vi "Resistance Test_ver2_3.vi"(0 "DMM ref in":refnum<visa-resource-name>, 1 "Measure\nMax Voltage":dbl=100.0, 2 "Resistance Test REF":refnum<vi>, 3 "Resistance Test Stop REF":refnum<vi>, 5 "PSU setting":T1, 7 "Channel  Count":i32, 9 "ESP32 ref in":refnum<visa-resource-name>="COM4", 11 "ESP32 error in":errorcluster, 12 "Wait Current Stable Period":u32, 13 "Manual Trigger Delay (1 s)":dbl=1.0, 14 "Current Sense \nResitance Array":dbl[](array[numeric])) -> (10 "ESP32 ref out":refnum<visa-resource-name>, 15 "ESP32 error out":errorcluster)   [LabVIEW 2023]
uses:
  <instrlib>/Agilent 3446X Series/Agilent 3446X Series.lvlib
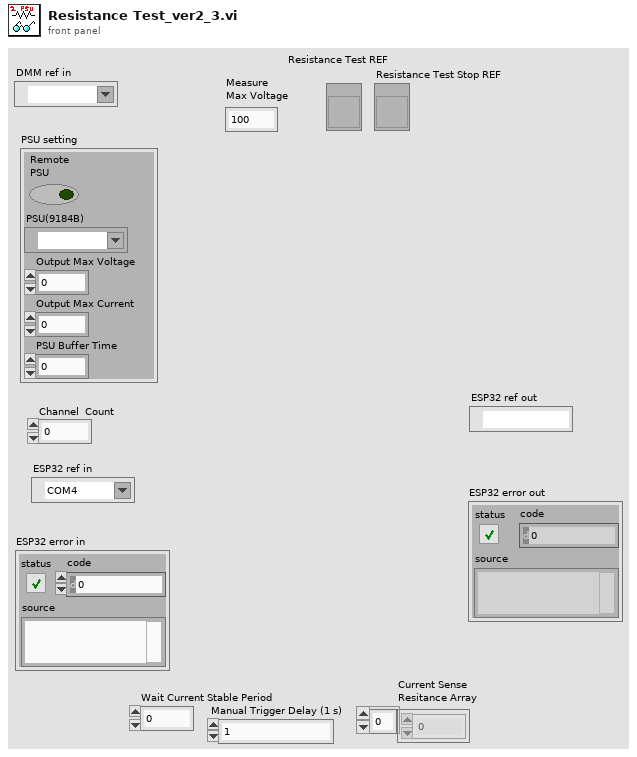
[diagram p1: front panel]
types:
  T1 = cluster{"Remote\nPSU":bool, "PSU(9184B)":refnum<visa-resource-name>, "Output Max Voltage":dbl, "Output Max Current":dbl, "PSU Buffer Time":u32}
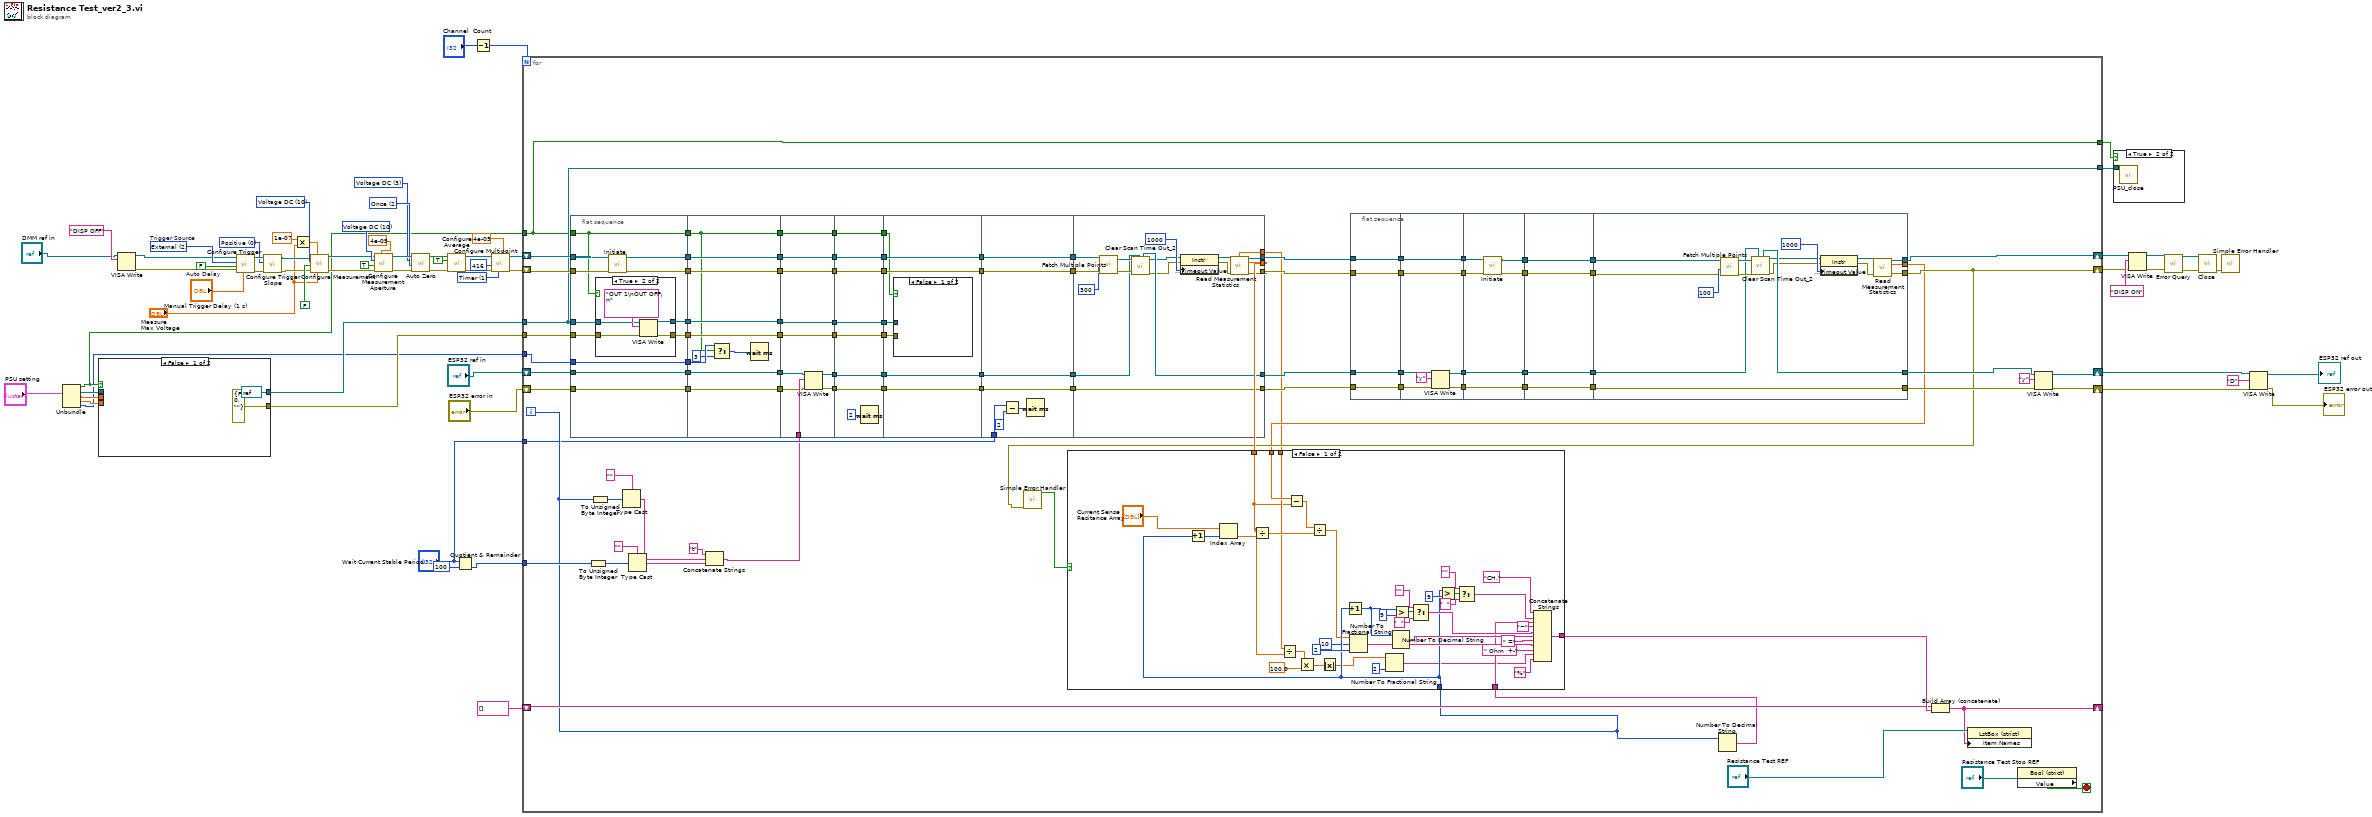
[diagram p0: block diagram]
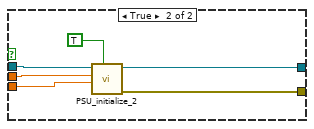
[diagram p3: hidden frame]
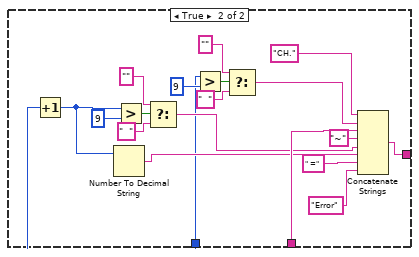
[diagram p4: hidden frame]
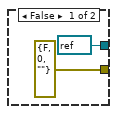
[diagram p5: hidden frame]
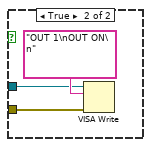
[diagram p6: hidden frame]
diagram:
  w28 = 0 items=["Positive", "Negative"] ("Trigger Edge (1: Negative)")
  w26 = 2 items=["Immediate", "Software (Bus)", "External"]  # Trigger Source
  w27 = FALSE  # Auto Delay
  w34 = 10 items=["Continuity", "Current AC", "Current DC", "Diode", "Frequency", "Resistance 4-wire", "Period", "Resistance 2-wire", "Temperature", "Voltage AC", "Voltage DC", "Voltage DC Ratio", "Capacitance"] ("Measurement Function (10: Voltage DC)")
  w38 = 1 items=["Immediate", "Timer"] ("Sample Source (0: Immediate)")
  w45 = 3 items=["Current DC", "Resistance", "Temperature", "Voltage DC"] ("Zero Type (0: Current DC)")
  w46 = 2 items=["Disable", "Enable", "Once"] ("Auto Zero (1: Enable)")
  w42 = 10 items=["Continuity", "Current AC", "Current DC", "Diode", "Frequency", "Resistance 4-wire", "Period", "Resistance 2-wire", "Temperature", "Voltage AC", "Voltage DC", "Voltage DC Ratio", "Capacitance"] ("Measurement Function (0: Continuity)")
  n1 = Unbundle("PSU setting") -> ("Remote\nPSU"=w6:bool, "PSU(9184B)"=w10:refnum<visa-resource-name>, "Output Max Voltage"=w9:dbl, "Output Max Current"=w8:dbl, "PSU Buffer Time"=w3:u32)
  n2 = case shown="False" w6 {
    tunnel: w10 -> [_ w75]
    tunnel: w9 -> [_ w74]
    tunnel: w8 -> [_ w73]
    tunnel: [refnum<visa-resource-name> refnum ("VISA resource name out") w71] -> w7
    tunnel: [errorcluster {"status"=FALSE, "code"=0, "source"=""} ("error out") w70] -> w5
    frame False {
    }
    frame True {
      n3 = call "PSU_initialize_2.vi"("safe Mode?"=TRUE, "Current"=w73, "Voltage"=w74, "VISA resource name"=w75) -> ("error out"=w70:errorcluster, "VISA resource name out"=w71:refnum<visa-resource-name>)  [unwired: 6 in]
    }
  }
  n4 = VISA Write(VISA resource name="DMM ref in", write buffer="DISP OFF") -> (VISA resource name out=w14:refnum<visa-resource-name>, error out=w13:errorcluster)  [unwired: 1 in, 1 out]
  n5 = call <instrlib>:"Configure Trigger.vi"("Manual Trigger Delay (1 s)"="Manual Trigger Delay (1 s)", "error in (no error)"=w13, "Auto Delay (F:Disable)"=w27, "Trigger Source (0: Immediate)"=w26, "VISA resource name"=w14) -> ("error out"=w30:errorcluster, "VISA resource name out"=w29:refnum<visa-resource-name>)  [unwired: 1 in, 4 out]
  n6 = call <instrlib>:"Configure Trigger Slope.vi"("error in (no error)"=w30, "Trigger Edge (1: Negative)"=w28, "VISA resource name"=w29) -> ("error out"=w24:errorcluster, "VISA resource name out"=w25:refnum<visa-resource-name>)  [unwired: 7 in]
  n7 = Multiply(x=1e-07, y="Measure\nMax Voltage") -> (x*y=w35:dbl)
  n8 = call <instrlib>:"Configure Measurement.vi"("Manual Range (1)"="Measure\nMax Voltage", "Absolute Resolution (1E-6)"=w35, "error in (no error)"=w24, "Auto Range (T: Enable)"=FALSE, "Measurement Function (10: Voltage DC)"=w34, "VISA resource name"=w25) -> ("error out"=w31:errorcluster, "VISA resource name out"=w32:refnum<visa-resource-name>)  [unwired: 4 out]
  n9 = call <instrlib>:"Configure Measurement Aperture.vi"("Aperture Time (0.1s)"=4e-05, "error in (no error)"=w31, "Enable Aperture (F: Disable)"=TRUE, "Measurement Function (0: Continuity)"=w42, "VISA resource name"=w32) -> ("error out"=w49:errorcluster, "VISA resource name out"=w48:refnum<visa-resource-name>)  [unwired: 5 in]
  n10 = call <instrlib>:"Auto Zero.vi"("error in (no error)"=w49, "Auto Zero (1: Enable)"=w46, "Zero Type (0: Current DC)"=w45, "VISA resource name"=w48) -> ("error out"=w51:errorcluster, "VISA resource name out"=w50:refnum<visa-resource-name>)  [unwired: 6 in]
  n11 = call <instrlib>:"Configure Average.vi"("error in (no error)"=w51, "Enable Statistics (F: Disable)"=TRUE, "VISA resource name"=w50) -> ("error out"=w40:errorcluster, "VISA resource name out"=w41:refnum<visa-resource-name>)  [unwired: 7 in]
  n12 = Quotient & Remainder(x="Wait Current Stable Period", y=100) -> (floor(x/y)=w20:u32)  [unwired: 1 out]
  n13 = Decrement(x="Channel  Count") -> (x-1=w18:i32)
  n14 = call <instrlib>:"Configure Multipoint.vi"("Sample Interval (1 Second)"=4e-05, "Sample Source (0: Immediate)"=w38, "error in (no error)"=w40, "Sample Count (1)"=416, "VISA resource name"=w41) -> ("error out"=w22:errorcluster, "VISA resource name out"=w23:refnum<visa-resource-name>)  [unwired: 2 in, 3 out]
  n15 = for {
    N: w18 -> [_]
    shift-right: [w128] -> w53
    shift-left: "ESP32 ref in" -> [w153]
    shift-right: [w126] -> w19
    shift-left: "ESP32 error in" -> [w151]
    shift-right: [w124] -> w54
    shift-left: w22 -> [w157]
    shift-right: [w163] -> w55
    shift-left: w23 -> [w158]
    shift-right: [w164] -> _
    shift-left: string[] [] -> [w166]
    tunnel: w20 -> [w141]
    tunnel: "Wait Current Stable Period" -> [w132]
    tunnel: w7 -> [w77]
    tunnel: w6 -> [w76]
    tunnel: w5 -> [w104]
    tunnel: w3 -> [w102]
    tunnel: [w77] -> w2
    tunnel: [w76] -> w1
    i -> [w139]
    stop <- w168 stop-if-true
    n16 = flat-sequence {
      tunnel: w157 -> [w273]
      tunnel: w158 -> [w275]
      tunnel: [w274] -> w162
      tunnel: [w272] -> w161
      tunnel: [w271] -> w154
      tunnel: w153 -> [w271]
      tunnel: w151 -> [w270]
      tunnel: [w270] -> w150
      tunnel: w76 -> [w266]
      tunnel: w77 -> [w269]
      tunnel: w104 -> [w268]
      tunnel: [w267] -> w103
      tunnel: w102 -> [w267]
      tunnel: [w266] -> w101
      tunnel: [w265] -> w99
      tunnel: [w264] -> w97
      tunnel: [w292] -> w160
      tunnel: [w291] -> w159
      tunnel: w162 -> [w292]
      tunnel: w161 -> [w291]
      tunnel: w154 -> [w290]
      tunnel: [w290] -> w152
      tunnel: w150 -> [w289]
      tunnel: [w289] -> w149
      tunnel: w103 -> [w288]
      tunnel: w101 -> [w283]
      tunnel: [w285] -> w100
      tunnel: w99 -> [w285]
      tunnel: [w284] -> w98
      tunnel: w97 -> [w284]
      tunnel: [w283] -> w82
      tunnel: w160 -> [w302]
      tunnel: [w302] -> w90
      tunnel: w159 -> [w301]
      tunnel: [w301] -> w92
      tunnel: w152 -> [w300]
      tunnel: w149 -> [w298]
      tunnel: w125 -> [w299]
      tunnel: [w297] -> w88
      tunnel: [w296] -> w86
      tunnel: w100 -> [w294]
      tunnel: w98 -> [w293]
      tunnel: [w295] -> w83
      tunnel: w82 -> [w295]
      tunnel: [w294] -> w81
      tunnel: [w293] -> w78
      tunnel: w92 -> [w310]
      tunnel: [w310] -> w91
      tunnel: w90 -> [w309]
      tunnel: [w309] -> w89
      tunnel: w88 -> [w308]
      tunnel: [w308] -> w87
      tunnel: w86 -> [w307]
      tunnel: [w307] -> w85
      tunnel: [w305] -> w84
      tunnel: w83 -> [w305]
      tunnel: w81 -> [w304]
      tunnel: [w304] -> w80
      tunnel: [w303] -> w79
      tunnel: w78 -> [w303]
      tunnel: w91 -> [w317]
      tunnel: [w317] -> w96
      tunnel: w89 -> [w316]
      tunnel: [w316] -> w95
      tunnel: w87 -> [w315]
      tunnel: [w315] -> w94
      tunnel: w85 -> [w314]
      tunnel: [w314] -> w93
      tunnel: w84 -> [w313]
      tunnel: w80 -> [w312]
      tunnel: w79 -> [w311]
      tunnel: w96 -> [w327]
      tunnel: [w327] -> w136
      tunnel: w95 -> [w326]
      tunnel: [w326] -> w135
      tunnel: w94 -> [w325]
      tunnel: [w325] -> w134
      tunnel: w93 -> [w324]
      tunnel: [w324] -> w133
      tunnel: w132 -> [w322]
      tunnel: [w341] -> w155
      tunnel: [w342] -> w156
      tunnel: w136 -> [w344]
      tunnel: w135 -> [w343]
      tunnel: [w334] -> w137
      tunnel: w134 -> [w335]
      tunnel: [w339] -> w131
      tunnel: w133 -> [w339]
      tunnel: [w338] -> w138
      tunnel: [w328] -> w105
      frame #0 {
        n17 = case shown="True" w266 {
          tunnel: w269 -> [_ w281]
          tunnel: w268 -> [_ w280]
          tunnel: [refnum<visa-resource-name> refnum ("VISA resource name out") w279] -> w265
          tunnel: [errorcluster {"status"=FALSE, "code"=0, "source"=""} ("error out") w278] -> w264
          frame False {
          }
          frame True {
            n18 = VISA Write(VISA resource name=w281, write buffer="OUT 1\nOUT OFF\n", error in (no error)=w280) -> (VISA resource name out=w279:refnum<visa-resource-name>, error out=w278:errorcluster)  [unwired: 1 out]
          }
        }
        n19 = call <instrlib>:"Initiate.vi"("error in (no error)"=w273, "VISA resource name"=w275) -> ("error out"=w272:errorcluster, "VISA resource name out"=w274:refnum<visa-resource-name>)  [unwired: 8 out]
      }
      frame #1 {
        n20 = Select(t=w288, s=w283, f=u32 3) -> (s? t:f=w286:u32)
        n21 = Wait (ms)(milliseconds to wait=w286) -> ()  [unwired: 1 out]
      }
      frame #2 {
        n22 = VISA Write(VISA resource name=w300, write buffer=w299, error in (no error)=w298) -> (VISA resource name out=w297:refnum<visa-resource-name>, error out=w296:errorcluster)  [unwired: 1 out]
      }
      frame #3 {
        n23 = Wait (ms)(milliseconds to wait=u32 2) -> ()  [unwired: 1 out]
      }
      frame #4 {
        n24 = case shown="False" w313 {
          tunnel: w312 -> [_ w319]
          tunnel: w311 -> [_ w318]
          frame False {
          }
          frame True {
            n25 = VISA Write(VISA resource name=w319, write buffer="OUT 1\nOUT ON\n", error in (no error)=w318) -> ()  [unwired: 3 out]
          }
        }
      }
      frame #5 {
        n26 = Subtract(x=w322, y=u32 2) -> (x-y=w323:u32)
        n27 = Wait (ms)(milliseconds to wait=w323) -> ()  [unwired: 1 out]
      }
      frame #6 {
        n28 = call <instrlib>:"Fetch Multiple Points.vi"("error in (no error)"=w344, "Timeout (10000 ms)"=300, "VISA resource name"=w343) -> ("error out"=w336:errorcluster, "VISA resource name out"=w337:refnum<visa-resource-name>)  [unwired: 1 in, 6 out]
        n29 = call "Clear Scan Time Out_2.vi"("ESP32 ref"=w335, "error in (no error)"=w336, "VISA Refnum in"=w337) -> ("error out"=w331:errorcluster, "VISA Refnum out"=w332:refnum<visa-resource-name>, "ESP32 ref out"=w334:refnum<visa-resource-name>)  [unwired: 4 in, 2 out]
        n30 = property class="Instr"(reference=w332, error in=w331, "General Settings:Timeout Value"=u32 1000) -> (reference out=w330:refnum<visa-resource-name>, error out=w329:errorcluster)
        n31 = call <instrlib>:"Read Measurement Statistics.vi"("VISA resource name"=w330, "error in (no error)"=w329) -> ("Standard Deviation"=w328:dbl, "VISA resource name out"=w342:refnum<visa-resource-name>, "Arithmetic Mean"=w338:dbl, "error out"=w341:errorcluster)  [unwired: 6 in, 4 out]
      }
    }
    n32 = To Unsigned Byte Integer(number=w141) -> (unsigned 8bit integer=w145:u8)
    n33 = To Unsigned Byte Integer(number=w139) -> (unsigned 8bit integer=w142:u8)
    n34 = Type Cast(type="" ("string"), x=w142) -> (*(type *) &x=w143:string)
    n35 = Type Cast(type="" ("string"), x=w145) -> (*(type *) &x=w144:string)
    n36 = Concatenate Strings("t" ("data in"), w143, w144) -> (w125:string)
    n37 = call <vilib>:"Simple Error Handler.vi"("error in (no error)"=w124) -> ("error?"=w123:bool)  [unwired: 4 in, 4 out]
    n38 = flat-sequence {
      tunnel: w131 -> [w170]
      tunnel: w137 -> [w171]
      tunnel: w155 -> [w172]
      tunnel: w156 -> [w173]
      tunnel: [w173] -> w122
      tunnel: [w172] -> w121
      tunnel: [w171] -> w120
      tunnel: [w170] -> w119
      tunnel: [w180] -> w118
      tunnel: [w179] -> w117
      tunnel: [w177] -> w116
      tunnel: [w174] -> w115
      tunnel: w122 -> [w180]
      tunnel: w121 -> [w179]
      tunnel: w120 -> [w178]
      tunnel: w119 -> [w175]
      tunnel: w118 -> [w184]
      tunnel: w117 -> [w183]
      tunnel: [w182] -> w114
      tunnel: w116 -> [w186]
      tunnel: [w186] -> w113
      tunnel: w115 -> [w185]
      tunnel: [w185] -> w112
      tunnel: [w181] -> w111
      tunnel: w114 -> [w190]
      tunnel: [w190] -> w110
      tunnel: w113 -> [w189]
      tunnel: [w189] -> w109
      tunnel: w112 -> [w188]
      tunnel: [w188] -> w108
      tunnel: w111 -> [w187]
      tunnel: [w187] -> w107
      tunnel: [w206] -> w106
      tunnel: [w204] -> w163
      tunnel: [w203] -> w124
      tunnel: [w199] -> w129
      tunnel: w110 -> [w191]
      tunnel: w109 -> [w200]
      tunnel: w108 -> [w193]
      tunnel: [w193] -> w127
      tunnel: w107 -> [w192]
      frame #0 {
      }
      frame #1 {
        n39 = VISA Write(VISA resource name=w178, write buffer="y", error in (no error)=w175) -> (VISA resource name out=w177:refnum<visa-resource-name>, error out=w174:errorcluster)  [unwired: 1 out]
      }
      frame #2 {
        n40 = call <instrlib>:"Initiate.vi"("error in (no error)"=w183, "VISA resource name"=w184) -> ("error out"=w182:errorcluster, "VISA resource name out"=w181:refnum<visa-resource-name>)  [unwired: 8 out]
      }
      frame #3 {
      }
      frame #4 {
        n41 = call <instrlib>:"Fetch Multiple Points.vi"("error in (no error)"=w191, "Timeout (10000 ms)"=100, "VISA resource name"=w192) -> ("error out"=w201:errorcluster, "VISA resource name out"=w202:refnum<visa-resource-name>)  [unwired: 1 in, 6 out]
        n42 = call "Clear Scan Time Out_2.vi"("ESP32 ref"=w200, "error in (no error)"=w201, "VISA Refnum in"=w202) -> ("error out"=w194:errorcluster, "VISA Refnum out"=w195:refnum<visa-resource-name>, "ESP32 ref out"=w199:refnum<visa-resource-name>)  [unwired: 4 in, 2 out]
        n43 = property class="Instr"(reference=w195, error in=w194, "General Settings:Timeout Value"=u32 1000) -> (reference out=w197:refnum<visa-resource-name>, error out=w196:errorcluster)
        n44 = call <instrlib>:"Read Measurement Statistics.vi"("VISA resource name"=w197, "error in (no error)"=w196) -> ("VISA resource name out"=w204:refnum<visa-resource-name>, "Arithmetic Mean"=w206:dbl, "error out"=w203:errorcluster)  [unwired: 6 in, 5 out]
      }
    }
    n45 = Number To Decimal String(number=w139) -> (decimal integer string=w140:string)  [unwired: 1 in]
    n46 = case shown="False" w123 {
      tunnel: [w239 w258] -> w167
      tunnel: w140 -> [w222 w255]
      tunnel: w106 -> [w210 _]
      tunnel: w139 -> [w223 w246]
      tunnel: w138 -> [w207 _]
      tunnel: w105 -> [w208 _]
      frame False {
        n47 = Increment(x=w223) -> (x+1=w227:i32)
        n48 = Index Array(array="Current Sense \nResitance Array", index=w227) -> (element=w221:dbl)
        n49 = Divide(x=w207, y=w221) -> (x/y=w219:dbl)
        n50 = Divide(x=w208, y=w207) -> (x/y=w216:dbl)
        n51 = Subtract(x=w210, y=w207) -> (x-y=w220:dbl)
        n52 = Multiply(x=w216, y=100.0) -> (x*y=w213:dbl)
        n53 = Divide(x=w220, y=w219) -> (x/y=w218:dbl)
        n54 = Absolute Value(x=w213) -> (abs(x)=w209:dbl)
        n55 = Increment(x=w223) -> (x+1=w230:i32)
        n56 = Number To Fractional String(number=w218, width (-)=i16 10, precision (6)=i16 2) -> (F-format string=w225:string)  [unwired: 1 in]
        n57 = Number To Fractional String(number=w209, precision (6)=i16 2) -> (F-format string=w212:string)  [unwired: 2 in]
        n58 = Number To Decimal String(number=w230) -> (decimal integer string=w229:string)  [unwired: 1 in]
        n59 = Greater?(x=w230, y=9) -> (0:w234:bool)
        n60 = Select(t="" ("string"), s=w234, f="  " ("string")) -> (s? t:f=w231:string)
        n61 = Greater?(x=w223, y=9) -> (0:w242:bool)
        n62 = Select(t="" ("string"), s=w242, f="  " ("string")) -> (s? t:f=w237:string)
        n63 = Concatenate Strings("CH." ("string"), w237, w222, "~" ("string"), w231, w229, " =" ("string"), w225, " Ohm  +-" ("string"), w212, "%" ("string")) -> (w239:string)
      }
      frame True {
        n64 = Increment(x=w246) -> (x+1=w248:i32)
        n65 = Number To Decimal String(number=w248) -> (decimal integer string=w247:string)  [unwired: 1 in]
        n66 = Greater?(x=w248, y=9) -> (0:w252:bool)
        n67 = Select(t="" ("string"), s=w252, f="  " ("string")) -> (s? t:f=w249:string)
        n68 = Greater?(x=w246, y=9) -> (0:w261:bool)
        n69 = Select(t="" ("string"), s=w261, f="  " ("string")) -> (s? t:f=w256:string)
        n70 = Concatenate Strings("CH." ("string"), w256, w255, "~" ("string"), w249, w247, " =" ("string"), "Error" ("string")) -> (w258:string)
      }
    }
    n71 = Build Array (concatenate)(w166, w167) -> (w164:string[])
    n72 = property class="LstBox (strict)"(reference="Resistance Test REF", "Item Names"=w164) -> ()  [unwired: 1 in, 2 out]
    n73 = property class="Bool (strict)"(reference="Resistance Test Stop REF") -> ("Value"=w168:bool)  [unwired: 1 in, 2 out]
    n74 = VISA Write(VISA resource name=w129, write buffer="y", error in (no error)=w127) -> (VISA resource name out=w128:refnum<visa-resource-name>, error out=w126:errorcluster)  [unwired: 1 out]
  }
  n75 = case shown="True" w1 {
    tunnel: w2 -> [_ w345]
    frame False {
    }
    frame True {
      n76 = call "PSU_close.vi"("VISA resource name"=w345) -> ()  [unwired: 11 in]
    }
  }
  n77 = VISA Write(VISA resource name=w55, write buffer="DISP ON", error in (no error)=w54) -> (VISA resource name out=w62:refnum<visa-resource-name>, error out=w61:errorcluster)  [unwired: 1 out]
  n78 = call <instrlib>:"Error Query.vi"("error in (no error)"=w61, "VISA resource name"=w62) -> ("error out"=w67:errorcluster, "VISA resource name out"=w66:refnum<visa-resource-name>)  [unwired: 8 out]
  n79 = call <instrlib>:"Close.vi"("error in (no error)"=w67, "VISA resource name"=w66) -> ("error out"=w65:errorcluster)  [unwired: 9 out]
  n80 = call <vilib>:"Simple Error Handler.vi"("error in (no error)"=w65) -> ()  [unwired: 1 in, 8 out]
  n81 = VISA Write(VISA resource name=w53, write buffer="D" ("data in"), error in (no error)=w19) -> (VISA resource name out=→"ESP32 ref out":refnum<visa-resource-name>, error out=→"ESP32 error out":errorcluster)  [unwired: 1 out]
